vi "PhidgetGetHubPort.vi"(8 "error in":errorcluster, 11 "Device In":u64) -> (0 "error out":errorcluster, 2 "Hub Port":i32, 3 "Device Out":u64)   [LabVIEW 2012, in "Phidget Common.lvlib"]
doc: "${HubPort:Header}"
uses:
  <instrlib>/Phidgets/Phidget Common/Phidget Common.lvlib
  phidget22.dll
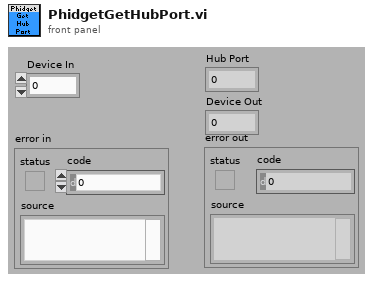
[diagram p1: front panel]
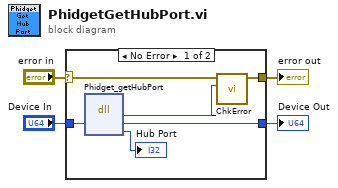
[diagram p0: block diagram]
diagram:
  n1 = case shown="No Error" "error in" {
    selector: "error in" -> [w7 w12]
    tunnel: [w5 w12] -> w3
    tunnel: [w10 w11] -> w2
    tunnel: "Device In" -> [w9 w11]
    frame No Error {
      n2 = dll-call lib="phidget22.*" fn="Phidget_getHubPort"("phid"=w9) -> ("return type"=w6:i32, "phid"=w10:u64, "port"=→"Hub Port":i32)  [unwired: 4 in, 2 out]
      n3 = call <instrlib>:"_ChkError.vi"("Return Code"=w6, "error in (no error)"=w7) -> ("error out"=w5:errorcluster)  [unwired: 9 in]
    }
    frame Error {
    }
  }
  "error out" <- w3
  "Device Out" <- w2
